vi "To Waveform.vi"(8 "error in (no error)":errorcluster, 11 "SensorData in":refnum<class "SensorData.lvclass">) -> (0 "error out":errorcluster, 2 "Waveform Graph":waveform(dbl)(graph), 3 "SensorData out":refnum<class "SensorData.lvclass">)   [LabVIEW 2012, in "Sensor Definition.lvlib" / "SensorData.lvclass"]
uses:
  SensorData.lvclass
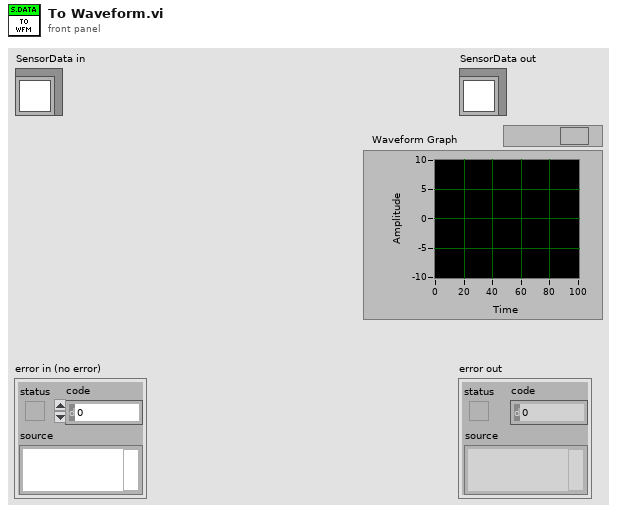
[diagram p1: front panel]
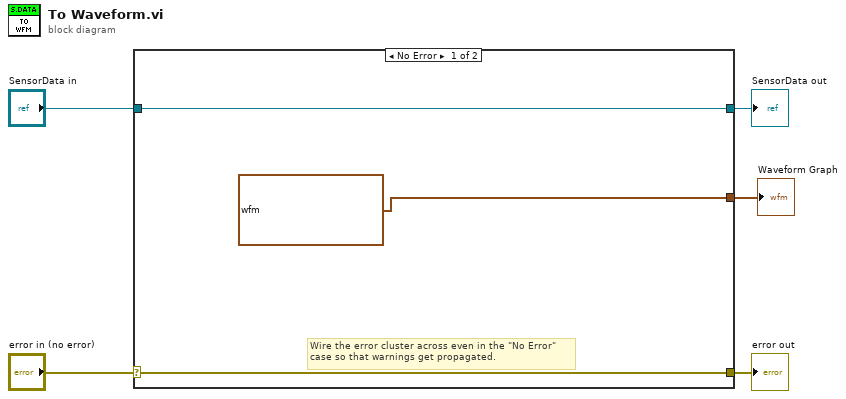
[diagram p0: block diagram]
diagram:
  n1 = case shown="No Error" "error in (no error)" {
    selector: "error in (no error)" -> [w7 w10]
    tunnel: [w7 w10] -> w4
    tunnel: [w8 w9] -> w2
    tunnel: "SensorData in" -> [w8 w9]
    tunnel: [waveform(dbl) {"t0"=timestamp(0 s since 1904-01-01), "dt"=1.0, "Y"=[]} ("Waveform") _] -> w1
    frame No Error {
      # "Wire the error cluster across even in the \"No Error\"\ncase so that warnings get propagated."
    }
    frame Error {
    }
  }
  "error out" <- w4
  "SensorData out" <- w2
  "Waveform Graph" <- w1
